vi "Init lib MPSSE.vi"(8 "error in (no error)":errorcluster) -> (0 "error out":errorcluster)   [LabVIEW 2018, in "libMPSSE-SPI.lvlib"]
doc: "FTDI_API void Init_libMPSSE(void);"
uses:
  libMPSSE-SPI.lvlib
  dll/libMPSSE.dll
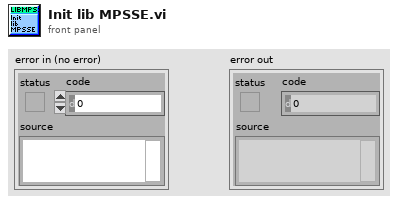
[diagram p1: front panel]
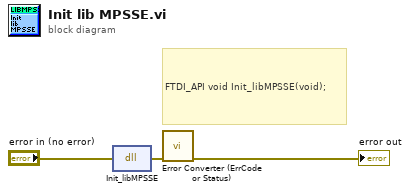
[diagram p0: block diagram]
diagram:
  # "FTDI_API void Init_libMPSSE(void);"
  n1 = dll-call lib="D:/LABVIEW/Examples - 32bit/FTDI/libMPSSE-SPI-LabVIEW-master/dll/libMPSSE.*" fn="Init_libMPSSE"(error in="error in (no error)") -> (error out=w2:errorcluster)  [unwired: 3 in, 1 out]
  n2 = call "Error Converter (ErrCode or Status).vi"("error in (no error)"=w2) -> ("error out"=→"error out":errorcluster)  [unwired: 10 in]
